vi "Main.vi"() -> ()   [LabVIEW 2026]
doc: "This Continuous Measurement sample project is based on the Queued Message Handler template.\n\nThe Event Handling Loop generates messages based on user interface actions.\n\nThe Message Handling Loop processes messages generated by the Event Handling Loop, or by other messages. There are also Acquisition and Logging message handling loop subVIs, and a chart updating loop."
uses:
  controls/VFD Notifier ctl.ctl
  Settings/Settings.ctl
  Acquisition/Hardware Configuration.ctl
  controls/Durability Test Conditions.ctl
  Logging/Logging Configuration.ctl
  controls/UI Data.ctl
  controls/UI State.ctl
  controls/NotifierAndDataQueue.ctl
  controls/WaveformChartData.ctl
  controls/Abort.vi
  controls/TestCaseTimer.vi
  support/Message Queue/Enqueue Message (Single).vi
  support/Message Queue/Enqueue Message (Array).vi
  <vilib>/Utility/error.llb/Error Cluster From Error Code.vi
  <vilib>/ErrorRing/Error Ring.xnode
  Acquisition/Acquisition.lvlib
  Logging/Logging.lvlib
  Settings/Settings.lvlib
  support/User Event - Stop/User Event - Stop.lvlib
  support/Message Queue/Message Queue.lvlib
  Control/Control.lvlib
panel:
  out "Live Pulley Ratio":dbl format="%#_2g"
  out "Calculated Pulley Ratio":dbl format="%#_2g"
  out "Fault Messages":string[](array[string])
  out "VFD Fault?":bool
  out "Speed (RPM)":dbl
  out "Current (A)":dbl
  out "Voltage (V)":dbl
  in  "Cluster":T1={"Voltage"=0.0, "Current"=0.0, "Motor Speed"=0.0, "Fault"=TRUE, "Fault Messages"=[]}
  in  "Clear Chart":bool
  out "Waveform Chart":T2(graph)
  in  "Tab Control":enum32{"Benchmarking", "Durability"}(tab)
  out "RPM Ramp":bool
  out "Free Air Flow":bool
  out "Press Stable":bool
  out "Press Decay":bool
  out "Status Table":string[][](table)
  out "Test State Timer":dbl(slide) scale=0.0..60.0
  out "INTAKE VALVE POSITION":bool
  out "Air Flow (LPM)":dbl(knob) scale=0.0..100.0
  out "DUT VALVE POSITION":bool
  out "Ambent Temp (F)":dbl(slide) scale=0.0..300.0 scale format="%#_3f"
  out "DUT Motor Current (A)":dbl format="%#_3f"
  out "DUT Temp (F)":dbl(slide) scale=0.0..300.0
  out "DUT Pressure (psi)":dbl(knob) scale=0.0..-15.0
  out "Tank Pressure (psi)":dbl(knob) scale=0.0..-15.0
  out "Drive Motor RPM":dbl(knob) scale=0.0..6000.0 scale format="%#_4f"
  out "DUT Pulley RPM":dbl(knob) scale=0.0..6000.0
  out "Belt Monitor":bool
  out "Status":string
  in  "Exit":bool
  in  "Stop":bool
  in  "Start":bool
  in  "Current Cycle Count":u64
  in  "Tab Control":T3(tab)
  in  "Durability Config File Path":path=path "C:/Users/ROlechna/OneDrive - Dorman Products/Desktop/Book1.csv"
  in  "Motor RPM Target":u16=1000
  in  "Test Selection Box":string(combo)="Benchmarking"
  in  "SKU # or File Name":string
  in  "DUT Motor Direction":bool
  in  "DUT Motor Enable":bool
  in  "Tank Inlet Valve Toggle":bool
  in  "Tank Outlet Valve Toggle":bool
  in  "VFD Enable":bool
  in  "VFD Reset":bool
  # "M1V1-1 Vacuum Pump Tester"
  # "SYSTEM & DUT PROPERTIES"
  # "**Case Timeout = 60s**"
  # "VFD State"
  # "Slot 3 NI 9264"
  # "Benchmarking Test Results"
  # "Durabilty Test Status"
  # "SYSTEM RPM MONITORING"
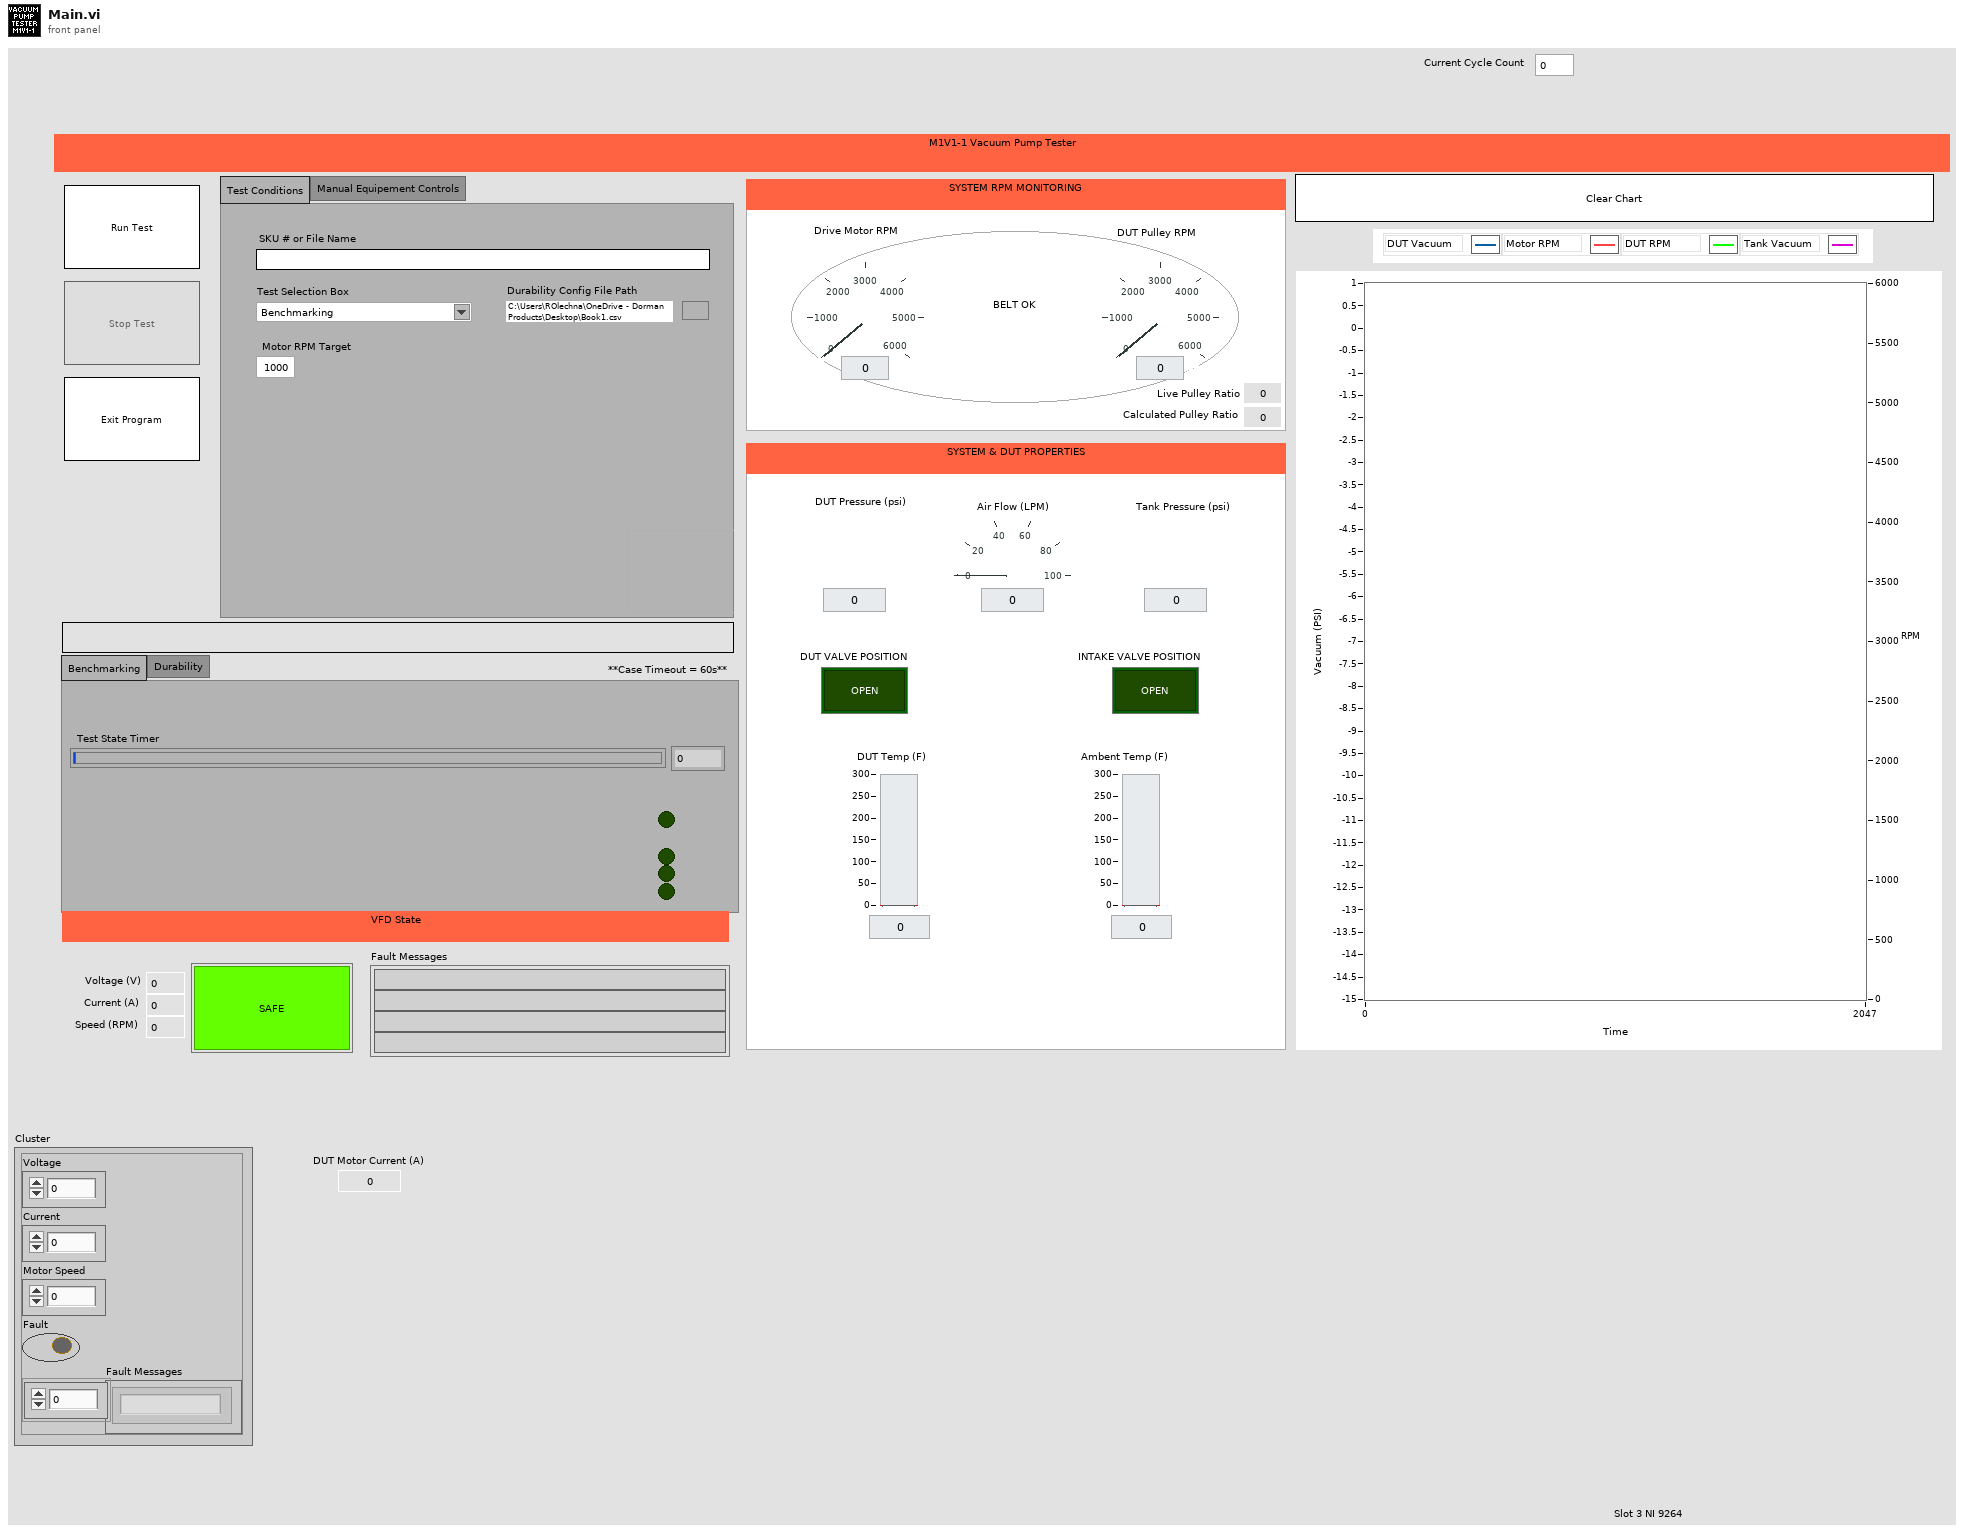
[diagram p1: front panel]
types:
  T1 = typedef "VFD Notifier ctl.ctl" = cluster{"Voltage":dbl, "Current":dbl, "Motor Speed":dbl, "Fault":bool, "Fault Messages":string[]}
  T2 = cluster{"DUT Vacuum":dbl, "Motor RPM":dbl, "DUT RPM":dbl, "Tank Vacuum":dbl}
  T3 = enum32{"Test Conditions", "Manual Equipement Controls"}
  T4 = typedef "NotifierAndDataQueue.ctl" = cluster{"Ai0":dbl, "Ai1":dbl, "Ai2":dbl, "Ai3":dbl, "Ai4":dbl, "Ai5":dbl, "Ai6":dbl, "Ai7":dbl, "Belt Slip?":bool, "P0.1":bool, "P0.2":bool, "P0.3":bool, "P0.4":bool, "P0.5":bool, "P0.6":bool, "P0.7":bool, "2D Numeric Data":dbl[][], "String 2":string, "String 1":string, "Waveform Chart Data":T5, "Live Pulley Ratio":dbl, "Data Table":string[][]}
  T5 = typedef "Settings.lvlib/WaveformChartData.ctl" = cluster{"DUT Vacuum":dbl, "Motor RPM":dbl, "DUT RPM":dbl, "Tank Vacuum":dbl}
  T6 = typedef "UI State.ctl" = enum16{"Idle", "Acquiring and Logging", "Waiting for Exit", "Waiting for Exit (Acq Stopped)", "Waiting for Exit (Log Stopped)", "Waiting for Stop", "Waiting for Stop (Acq Stopped)", "Waiting for Stop (Log Stopped)"}
  T7 = typedef "UI Data.ctl" = cluster{"Start Ref":refnum<vi>, "Trigger Ref":refnum<vi>, "Stop Ref":refnum<vi>, "Settings Ref":refnum<vi>, "Status Ref":refnum<vi>, "Exit Ref":refnum<vi>, "Data Ref":refnum<vi>}
  T8 = typedef "Settings.lvlib/Settings.ctl" = cluster{"Hardware Configuration":T9, "Logging Configuration":T11}
  T9 = typedef "Acquisition.lvlib/Hardware Configuration.ctl" = cluster{"Analog Out array":dbl[], "Initialize Flag":bool, "Saftey Table Display":refnum<vi>, "Torque&Force":waveform(dbl)[][], "Calibration Data":waveform(dbl)[], "2D":dbl[][], "Analog In Task":refnum<k21>, "Digital In Task":refnum<k21>, "Analog Out Task":refnum<k21>, "Digital Out Task":refnum<k21>, "Digital Out Array":bool[], "Current Cycle Count":refnum<vi>, "Cycle Count":u64, "Headers":string[], "Sweep Interval":u64, "Delay":u64, "TestConfigDisplay":refnum<vi>, "50psi Conversion":dbl[], "1245N15 Conversion":dbl[], "MX06F Conversion":dbl[], "# of Test Cycles":u64, "60psi Conversion":dbl[], "100psi Conversion":dbl[], "200psi Conversion":dbl[], "1000psi Conversion":dbl[], "2000psi Conversion":dbl[], "5000psi Conversion":dbl[], "MX09F Conversion":dbl[], "MX19F Conversion":dbl[], "DUT VALVE POSITION":refnum<vi>, "INTAKE VALVE POSITION":refnum<vi>, "Table Control":refnum<vi>, "Table Control":string[][], "Max Vacuum":dbl, "RPM Ramp Ref":refnum<vi>, "Free Air Flow Ref":refnum<vi>, "Press Stable Ref":refnum<vi>, "Press Decay Ref":refnum<vi>, "Pulley Ratio":dbl, "Calculated Pulley Ratio":refnum<vi>, "Durability Test Conditions":T10, "# of Durab Steps":dbl, "manual aquire timer":dbl, "Durability Test Conditions Initial":T10}
  T10 = typedef "Durability Test Conditions.ctl" = cluster{"Step #s":dbl[], "RPMs":dbl[], "Step Durations":dbl[], "Step Delays":dbl[], "Test Cycles":dbl}
  T11 = typedef "Logging.lvlib/Logging Configuration.ctl" = cluster{"Log File Base Path":path, "TDMS File Reference":refnum<k34>, "File Name":string, "Headers To Write":string[]}
  T12 = typedef "Message Queue.lvlib/All Message Queues.ctl" = cluster{"UI":refnum<queue>, "Acquisition":refnum<queue>, "Logging":refnum<queue>, "Control":refnum<queue>, "VFD Control":refnum<queue>}
  T13 = cluster{"DUT Vacuum":dbl, "Motor RPM":dbl, "DUT RPM":dbl, "Tank Vacuum":dbl}[]
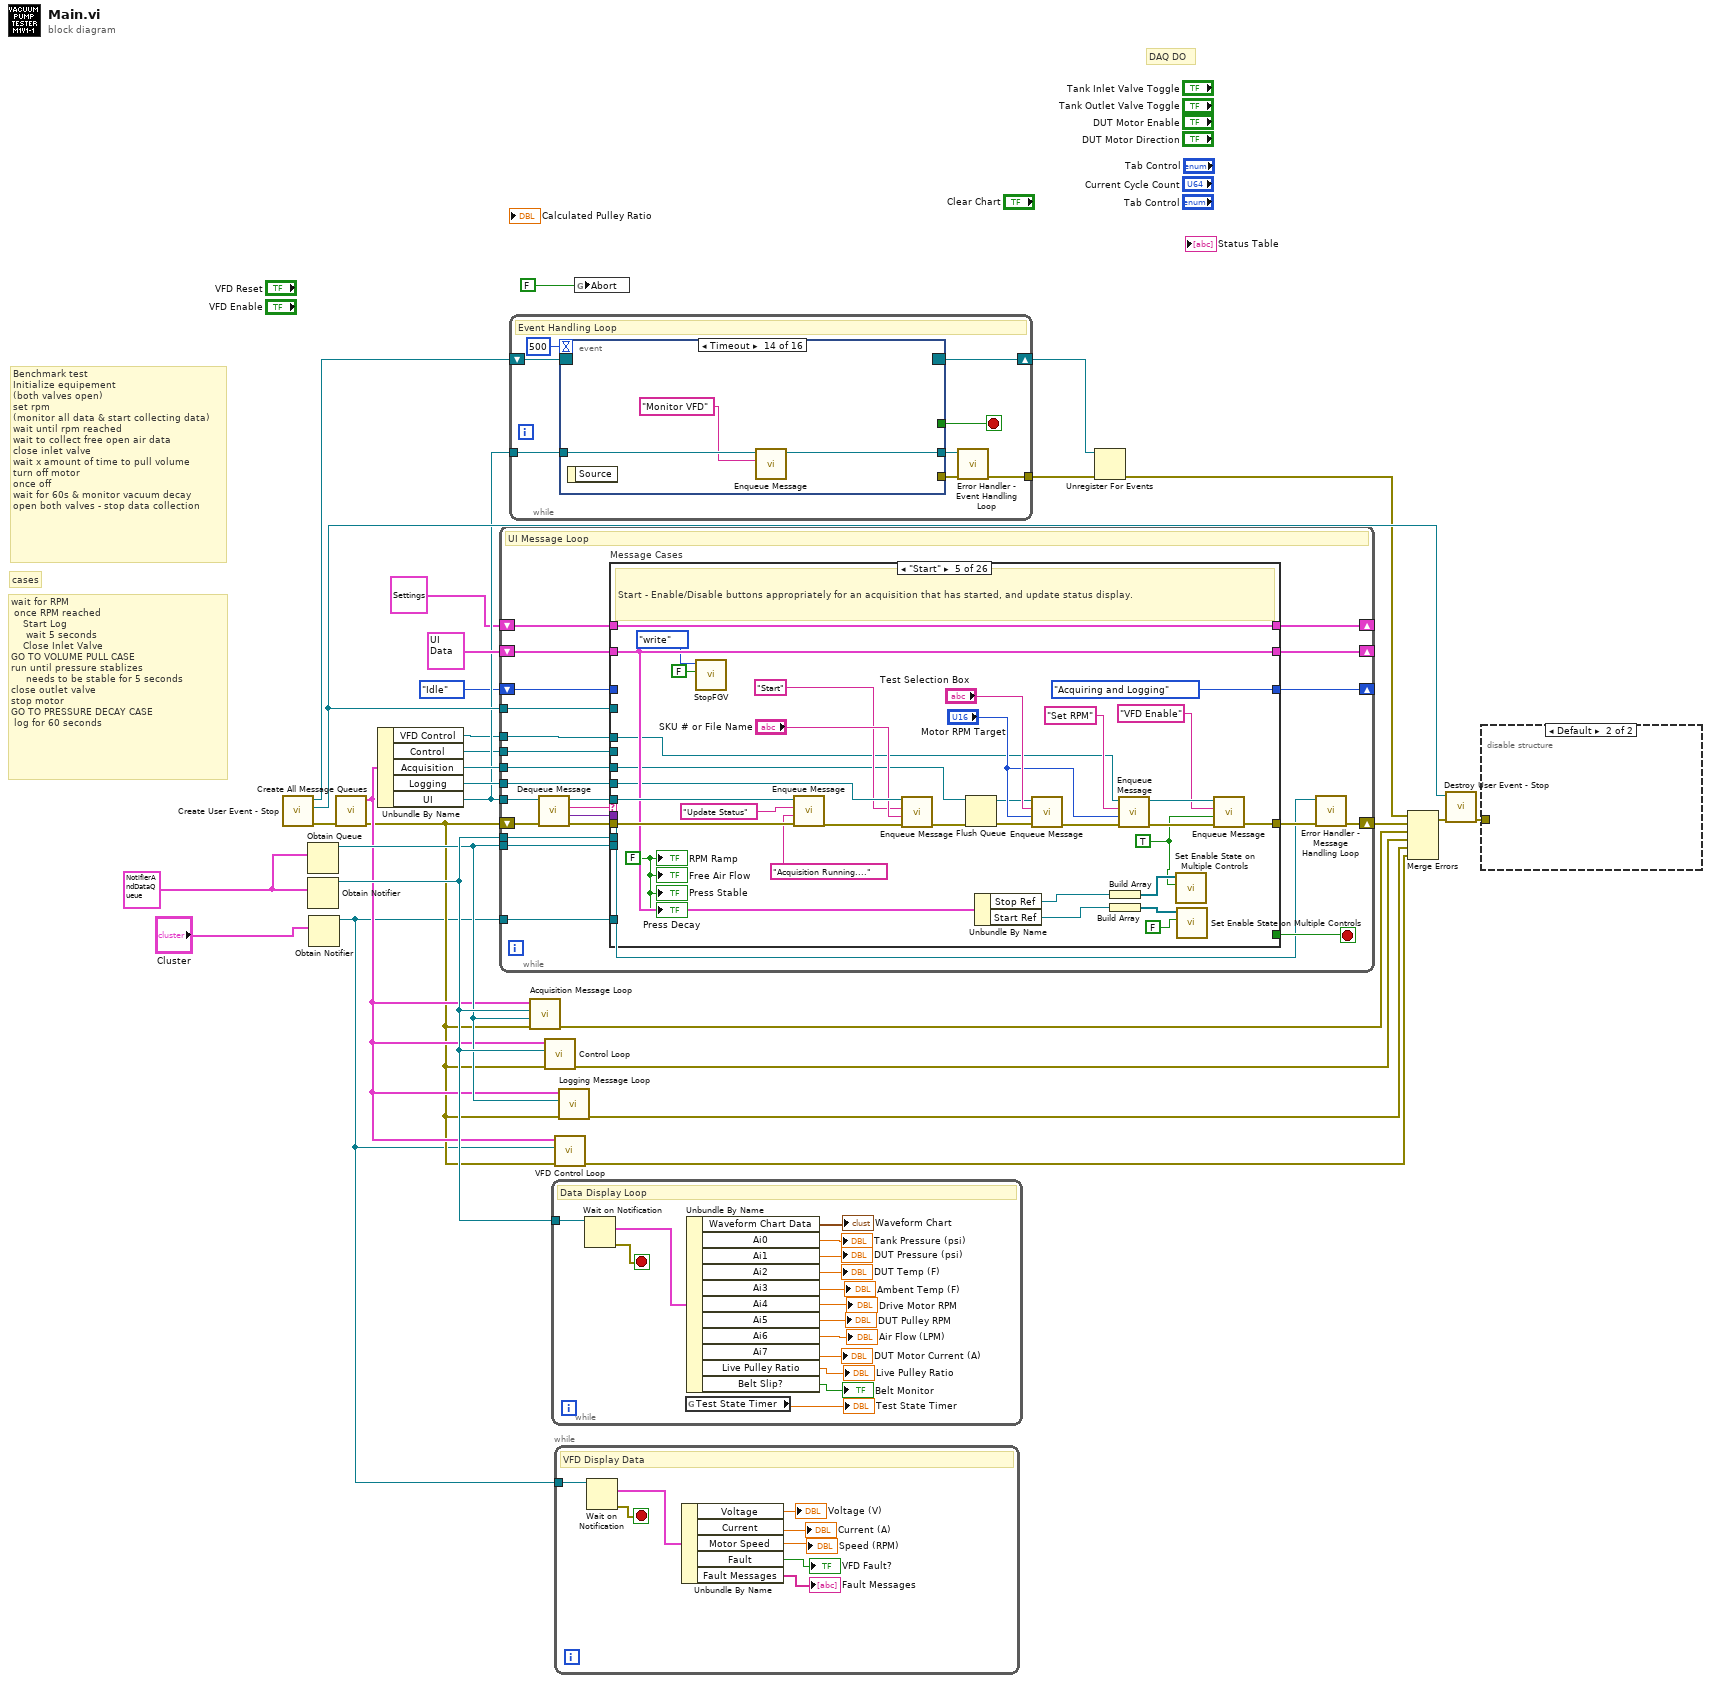
[diagram p0: block diagram]
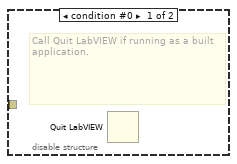
[diagram p2: hidden frame]
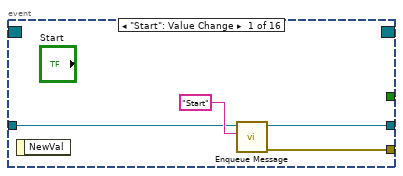
[diagram p3: hidden frame]
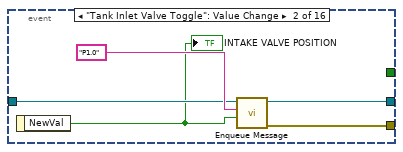
[diagram p4: hidden frame]
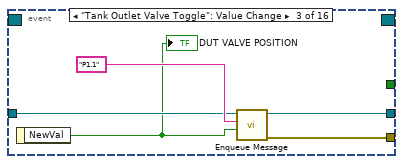
[diagram p5: hidden frame]
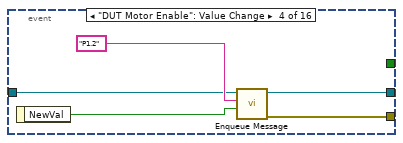
[diagram p6: hidden frame]
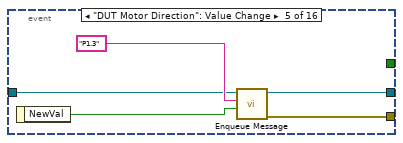
[diagram p7: hidden frame]
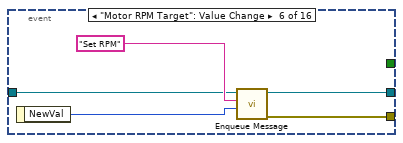
[diagram p8: hidden frame]
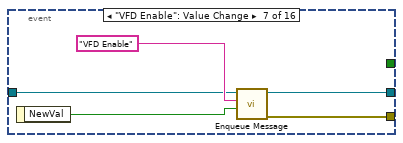
[diagram p9: hidden frame]
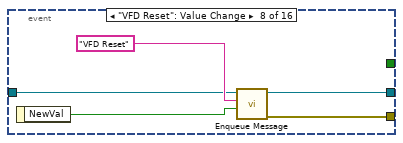
[diagram p10: hidden frame]
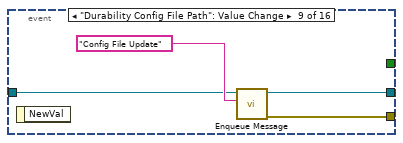
[diagram p11: hidden frame]
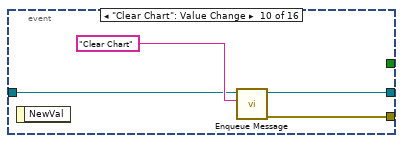
[diagram p12: hidden frame]
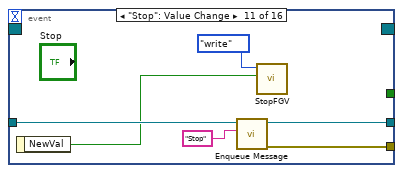
[diagram p13: hidden frame]
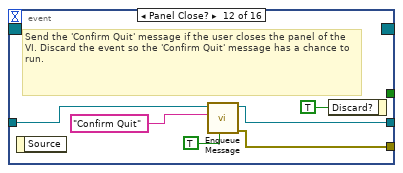
[diagram p14: hidden frame]
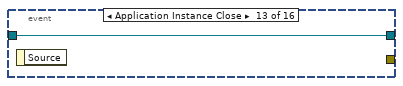
[diagram p15: hidden frame]
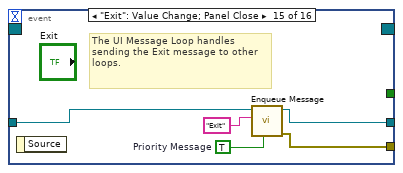
[diagram p16: hidden frame]
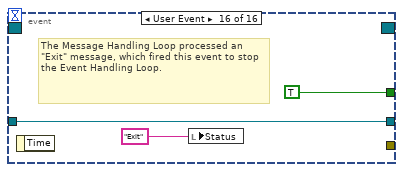
[diagram p17: hidden frame]
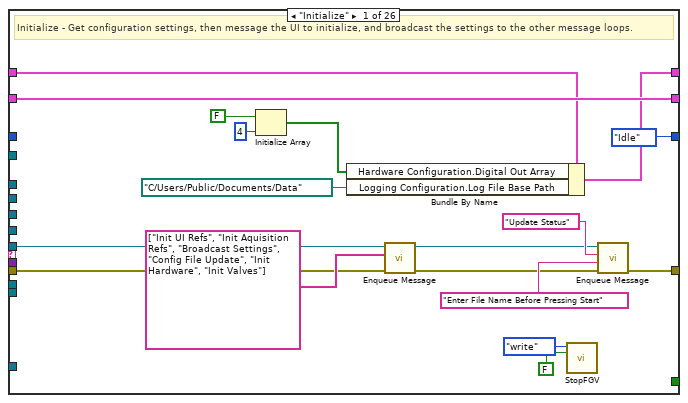
[diagram p18: hidden frame]
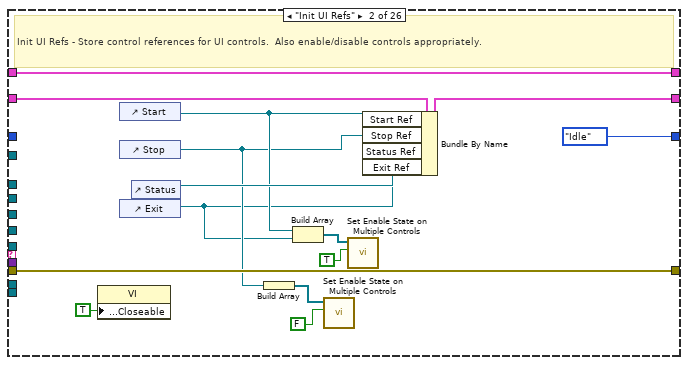
[diagram p19: hidden frame]
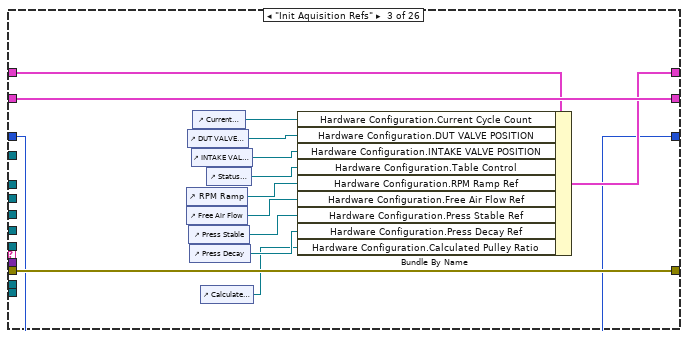
[diagram p20: hidden frame]
diagram:
  w8 = T4 {"Ai0"=0.0, "Ai1"=0.0, "Ai2"=0.0, "Ai3"=0.0, "Ai4"=0.0, "Ai5"=0.0, "Ai6"=0.0, "Ai7"=0.0, "Belt Slip?"=FALSE, "P0.1"=FALSE, "P0.2"=FALSE, "P0.3"=FALSE, "P0.4"=FALSE, "P0.5"=FALSE, "P0.6"=FALSE, "P0.7"=FALSE, "2D Numeric Data"=[], "String 2"="", "String 1"="", "Waveform Chart Data"={"DUT Vacuum"=0.0, "Motor RPM"=0.0, "DUT RPM"=0.0, "Tank Vacuum"=0.0}, "Live Pulley Ratio"=0.0, "Data Table"=[]} ("Waveform")
  # "cases"
  # "wait for RPM\n once RPM reached\n    Start Log\n     wait 5 seconds\n    Close Inlet Valve\nGO TO VOLUME PULL CASE\nrun until pressure stablizes\n     needs to be stable for 5 seconds\nclose outlet valve\nstop motor\nGO TO PRESSURE DECAY CASE\n log for 60 seconds"
  # "Benchmark test\nInitialize equipement\n(both valves open)\nset rpm\n(monitor all data & start collecting data)\nwait until rpm reached\nwait to collect free open air data\nclose inlet valve\nwait x amount of time to pull volume\nturn off motor\nonce off\nwait for 60s & monitor vacuum decay\nopen both valves - stop data collection"
  # "DAQ DO"
  n1 = call "Create User Event - Stop.vi"() -> ("error out"=w23:errorcluster, "User Event - Stop"=w25:refnum<user-event>, "Stop Event Registration Refnum"=w26:refnum<event-registration>)  [unwired: 9 in]
  n2 = Obtain Queue(element data type=w8) -> (queue out=w7:refnum<queue>)  [unwired: 4 in, 2 out]
  n3 = Obtain Notifier(notification data type=w8) -> (notifier out=w9:refnum<notifier>)  [unwired: 3 in, 2 out]
  n4 = Obtain Notifier(notification data type="Cluster") -> (notifier out=w1:refnum<notifier>)  [unwired: 3 in, 2 out]
  n5 = call "Create All Message Queues.vi"("error in (no error)"=w23) -> ("error out"=w5:errorcluster, "Message Queues out"=w6:T12)  [unwired: 9 in]
  n6 = Unbundle By Name(w6) -> ("VFD Control"=w3:refnum<queue>, "Control"=w14:refnum<queue>, "Acquisition"=w19:refnum<queue>, "Logging"=w18:refnum<queue>, "UI"=w17:refnum<queue>)
  n7 = while {
    tunnel: w17 -> [w46]
    tunnel: w25 -> [w51]
    shift-right: [w36] -> w29
    shift-left: w5 -> [w50]
    shift-right: [w45] -> _
    shift-left: T8 {"Hardware Configuration"={"Analog Out array"=[], "Initialize Flag"=FALSE, "Saftey Table Display"=refnum, "Torque&Force"=[], "Calibration Data"=[], "2D"=[], "Analog In Task"="", "Digital In Task"="", "Analog Out Task"="", "Digital Out Task"="", "Digital Out Array"=[], "Current Cycle Count"=refnum, "Cycle Count"=0, "Headers"=[], "Sweep Interval"=0, "Delay"=0, "TestConfigDisplay"=refnum, "50psi Conversion"=[], "1245N15 Conversion"=[], "MX06F Conversion"=[], "# of Test Cycles"=0, "60psi Conversion"=[], "100psi Conversion"=[], "200psi Conversion"=[], "1000psi Conversion"=[], "2000psi Conversion"=[], "5000psi Conversion"=[], "MX09F Conversion"=[], "MX19F Conversion"=[], "DUT VALVE POSITION"=refnum, "INTAKE VALVE POSITION"=refnum, "Table Control"=refnum, "Table Control"=[], "Max Vacuum"=0.0, "RPM Ramp Ref"=refnum, "Free Air Flow Ref"=refnum, "Press Stable Ref"=refnum, "Press Decay Ref"=refnum, "Pulley Ratio"=0.0, "Calculated Pulley Ratio"=refnum, "Durability Test Conditions"={"Step #s"=[], "RPMs"=[], "Step Durations"=[], "Step Delays"=[], "Test Cycles"=0.0}, "# of Durab Steps"=0.0, "manual aquire timer"=0.0, "Durability Test Conditions Initial"={"Step #s"=[], "RPMs"=[], "Step Durations"=[], "Step Delays"=[], "Test Cycles"=0.0}}, "Logging Configuration"={"Log File Base Path"=path "", "TDMS File Reference"=refnum, "File Name"="", "Headers To Write"=[]}} ("Settings") -> [w44]
    shift-right: [w42] -> _
    shift-left: T7 {"Start Ref"=refnum, "Trigger Ref"=refnum, "Stop Ref"=refnum, "Settings Ref"=refnum, "Status Ref"=refnum, "Exit Ref"=refnum, "Data Ref"=refnum} ("Measurement UI Controls") -> [w43]
    tunnel: w19 -> [w41]
    tunnel: w18 -> [w40]
    tunnel: w9 -> [w39]
    tunnel: w7 -> [w38]
    shift-right: [w33] -> _
    shift-left: UI_State."Idle" ("UI State") -> [w34]
    tunnel: w14 -> [w32]
    tunnel: w3 -> [w31]
    tunnel: w1 -> [w30]
    stop <- w52 stop-if-true
    # "UI Message Loop"
    n8 = call "Dequeue Message.vi"("error in (no error)"=w50, "Message Queue"=w46) -> ("error out"=w49:errorcluster, "Message Data"=w47:variant, "Message"=w48:string, "dup Message Queue"=w35:refnum<queue>)  [unwired: 6 in]
    n9 = case "Message Cases" shown="\"Start\"" w48 {
      selector: w48 -> [_ _ _ _ _ _ _ _ _ _ _ _ _ _ _ _ _ _ _ _ _ _ _ _ _ w420]
      tunnel: w35 -> [w66 _ _ _ w140 _ _ w161 _ _ _ _ _ w241 w251 w276 _ _ _ _ _ _ w360 w370 w408 _]
      tunnel: w49 -> [w65 w84 w98 w106 w139 w146 w155 w171 w179 w188 w197 w206 w215 w240 w253 w278 w306 w321 w329 w336 w341 w349 w364 w369 w413 _]
      tunnel: [w53 w84 w98 w107 w120 w149 w158 w173 w182 w191 w200 w209 w218 w224 w252 w277 w301 w315 w328 w335 w341 w348 w355 w368 w414 w421] -> w37
      tunnel: [_ _ _ _ _ _ _ _ _ _ _ _ _ _ _ _ _ _ _ _ _ _ _ _ TRUE _] -> w52
      tunnel: w47 -> [_ _ _ w105 _ w141 w150 _ w174 w183 w193 w202 w211 _ _ _ _ _ _ _ _ _ w363 _ _ _]
      tunnel: w51 -> [_ _ _ _ _ _ _ _ _ _ _ _ _ _ _ _ _ _ _ _ _ _ _ _ w412 _]
      tunnel: [w63 w83 w95 w102 w128 w148 w157 w172 w181 w190 w199 w208 w217 w239 w257 w282 w305 w323 w331 w338 w344 w353 w366 w373 w410 w423] -> w45
      tunnel: w44 -> [w54 w83 w96 w102 w128 w148 w157 w172 w181 w190 w199 w208 w217 w239 w257 w282 w305 w323 w331 w338 w344 w353 w366 w373 w410 w423]
      tunnel: w43 -> [w68 w82 w97 w101 w136 w147 w156 w165 w180 w189 w198 w207 w216 w236 w256 w281 w308 w322 w330 w337 w343 w352 w365 w372 w409 w422]
      tunnel: [w68 w81 w97 w101 w136 w147 w156 w165 w180 w189 w198 w207 w216 w236 w256 w281 w308 w322 w330 w337 w343 w352 w365 w372 w409 w422] -> w42
      tunnel: w41 -> [_ _ _ _ w108 _ _ w168 _ _ _ _ _ w222 _ _ w303 w320 _ _ _ w347 _ _ w401 _]
      tunnel: w40 -> [_ _ _ _ w130 _ _ _ _ _ _ _ _ w221 _ _ _ _ _ _ _ _ _ _ w400 _]
      tunnel: w39 -> [_ _ _ _ _ _ _ _ _ _ _ _ _ _ _ _ _ _ _ _ _ _ _ _ w407 _]
      tunnel: w38 -> [_ _ _ _ _ _ _ _ _ _ _ _ _ _ _ _ _ _ _ _ _ _ _ _ w404 _]
      tunnel: w34 -> [_ _ w94 w99 _ w143 w152 _ w176 w185 w194 w203 w212 w226 w255 w280 w307 w316 w324 w334 w342 w350 w354 w371 _ w419]
      tunnel: [UI_State."Idle" ("UI State") UI_State."Idle" ("UI State") w94 w99 UI_State."Acquiring and Logging" ("UI State") w143 w152 UI_State."Acquiring and Logging" ("UI State") w176 w185 w194 w203 w212 w225 w254 w279 w307 w316 w324 w334 w342 w350 w354 w367 UI_State."Idle" ("UI State") w419] -> w33
      tunnel: w32 -> [_ _ _ _ _ w142 w151 _ w175 w184 _ _ _ w223 _ _ w302 w318 w327 _ _ _ _ _ w402 _]
      tunnel: w31 -> [_ _ _ _ w112 _ _ _ _ _ w192 w201 w210 w219 _ _ _ _ _ w332 _ _ _ _ w398 _]
      tunnel: w30 -> [_ _ _ _ _ _ _ _ _ _ _ _ _ _ _ _ _ _ _ _ _ _ _ _ w395 _]
      frame "Initialize" {
        # "Initialize - Get configuration settings, then message the UI to initialize, and broadcast the settings to the other message loops."
        n10 = Initialize Array(FALSE, 4 ("dimension size")) -> (w57:bool[])
        n11 = Bundle By Name(cluster=w54, "Hardware Configuration.Digital Out Array"=w57, "Logging Configuration.Log File Base Path"=path "C:/Users/Public/Documents/Data") -> (w63:T8)
        n12 = call-poly "Enqueue Message.vi"("error in (no error)"=w65, "Message Array"=string[] ["Init UI Refs", "Init Aquisition Refs", "Broadcast Settings", "Config File Update", "Init Hardware", "Init Valves"] ("Message"), "Message Queue"=w66) -> ("error out"=w61:errorcluster, "dup Message Queue"=w62:refnum<queue>)  [unwired: 7 in]
        n13 = call "StopFGV.vi"("STOP"=FALSE, "Enum"=enum16{"init", "write", "read"}."write") -> ()  [unwired: 8 in, 2 out]
        n14 = call-poly "Enqueue Message.vi"("error in (no error)"=w61, "Message Data"="Enter File Name Before Pressing Start" ("Ready..."), "Message"="Update Status", "Message Queue"=w62) -> ("error out"=w53:errorcluster)  [unwired: 6 in, 1 out]
      }
      frame "Init UI Refs" {
        # "Init UI Refs - Store control references for UI controls.  Also enable/disable controls appropriately."
        n15 = property class="VI"("Front Panel.Closeable"=TRUE ("Front Panel Window:Closeable")) -> ()  [unwired: 2 in, 2 out]
        n16 = control-ref of="Start"() -> (w73:refnum<vi>)
        n17 = control-ref of="Stop"() -> (w72:refnum<vi>)
        n18 = control-ref of="Exit"() -> (w71:refnum<vi>)
        n19 = control-ref of="Status"() -> (w78:refnum<vi>)
        n20 = Build Array(w72) -> (w77:refnum<vi>[])
        n21 = Build Array(w73, w71) -> (w75:refnum<vi>[])
        n22 = call "Set Enable State on Multiple Controls.vi"("Enable?"=FALSE, "Controls"=w77) -> ()  [unwired: 10 in]
        n23 = call "Set Enable State on Multiple Controls.vi"("Enable?"=TRUE, "Controls"=w75) -> ()  [unwired: 10 in]
        n24 = Bundle By Name(cluster=w82, "Start Ref"=w73, "Stop Ref"=w72, "Status Ref"=w78, "Exit Ref"=w71) -> (w81:T7)
      }
      frame "Init Aquisition Refs" {
        n25 = control-ref of="RPM Ramp"() -> (w89:refnum<vi>)
        n26 = control-ref of="Free Air Flow"() -> (w88:refnum<vi>)
        n27 = control-ref of="DUT VALVE POSITION"() -> (w92:refnum<vi>)
        n28 = control-ref of="Press Stable"() -> (w87:refnum<vi>)
        n29 = control-ref of="Press Decay"() -> (w86:refnum<vi>)
        n30 = control-ref of="INTAKE VALVE POSITION"() -> (w91:refnum<vi>)
        n31 = control-ref of="Current Cycle Count"() -> (w93:refnum<vi>)
        n32 = control-ref of="Calculated Pulley Ratio"() -> (w85:refnum<vi>)
        n33 = control-ref of="Status Table"() -> (w90:refnum<vi>)
        n34 = Bundle By Name(cluster=w96, "Hardware Configuration.Current Cycle Count"=w93, "Hardware Configuration.DUT VALVE POSITION"=w92, "Hardware Configuration.INTAKE VALVE POSITION"=w91, "Hardware Configuration.Table Control"=w90, "Hardware Configuration.RPM Ramp Ref"=w89, "Hardware Configuration.Free Air Flow Ref"=w88, "Hardware Configuration.Press Stable Ref"=w87, "Hardware Configuration.Press Decay Ref"=w86, "Hardware Configuration.Calculated Pulley Ratio"=w85) -> (w95:T8)
      }
      frame "Update Status" {
        # "Update Display - Convert the message data to a string to display in the Status indicator."
        n35 = Variant To Data(error in=w106, type="", Variant=w105) -> (data=→"Status":string, error out=w103:errorcluster)
        n36 = Merge Errors(w103) -> (w107:errorcluster)
      }
      frame "Start" {
        w121 = FALSE
        w114 = TRUE ("Enable?")
        # "Start - Enable/Disable buttons appropriately for an acquisition that has started, and update status display."
        n37 = call "StopFGV.vi"("STOP"=FALSE, "Enum"=enum16{"init", "write", "read"}."write") -> ()  [unwired: 8 in, 2 out]
        n38 = call-poly "Enqueue Message.vi"("error in (no error)"=w139, "Message Data"="Acquisition Running...." ("Waiting for trigger"), "Message"="Update Status", "Message Queue"=w140) -> ("error out"=w131:errorcluster)  [unwired: 6 in, 1 out]
        n39 = call-poly "Enqueue Message.vi"("error in (no error)"=w131, "Message Data"="SKU # or File Name", "Message"="Start", "Message Queue"=w130) -> ("error out"=w111:errorcluster)  [unwired: 6 in, 1 out]
        n40 = Flush Queue(queue=w108, error in (no error)=w111) -> (queue out=w109:refnum<queue>, error out=w110:errorcluster)  [unwired: 1 out]
        n41 = Unbundle By Name(w136) -> ("Stop Ref"=w127:refnum<vi>, "Start Ref"=w132:refnum<vi>)
        n42 = call-poly "Enqueue Message.vi"("error in (no error)"=w110, "Message Data"="Motor RPM Target", "Message"="Test Selection Box", "Message Queue"=w109) -> ("error out"=w119:errorcluster)  [unwired: 6 in, 1 out]
        n43 = Build Array(w127) -> (w133:refnum<vi>[])
        n44 = Build Array(w132) -> (w134:refnum<vi>[])
        n45 = call-poly "Enqueue Message.vi"("error in (no error)"=w119, "Message Data"="Motor RPM Target", "Message"="Set RPM", "Message Queue"=w112) -> ("error out"=w118:errorcluster, "dup Message Queue"=w117:refnum<queue>)  [unwired: 6 in]
        n46 = call "Set Enable State on Multiple Controls.vi"("Enable?"=w114, "Controls"=w133) -> ()  [unwired: 10 in]
        n47 = call "Set Enable State on Multiple Controls.vi"("Enable?"=FALSE, "Controls"=w134) -> ()  [unwired: 10 in]
        n48 = call-poly "Enqueue Message.vi"("error in (no error)"=w118, "Message Data"=w114, "Message"="VFD Enable", "Message Queue"=w117) -> ("error out"=w120:errorcluster)  [unwired: 6 in, 1 out]
        "RPM Ramp" <- w121
        "Free Air Flow" <- w121
        "Press Stable" <- w121
        "Press Decay" <- w121
      }
      frame "P1.0" {
        # "Force Trigger - send a message to the Logging message loop to start logging."
        n49 = call-poly "Enqueue Message.vi"("error in (no error)"=w146, "Message Data"=w141, "Message"="P1.0", "Message Queue"=w142) -> ("error out"=w145:errorcluster)  [unwired: 6 in, 1 out]
        n50 = Merge Errors(w145) -> (w149:errorcluster)
      }
      frame "P1.1" {
        # "Force Trigger - send a message to the Logging message loop to start logging."
        n51 = call-poly "Enqueue Message.vi"("error in (no error)"=w155, "Message Data"=w150, "Message"="P1.1", "Message Queue"=w151) -> ("error out"=w154:errorcluster)  [unwired: 6 in, 1 out]
        n52 = Merge Errors(w154) -> (w158:errorcluster)
      }
      frame "Manual Acquire" {
        # "Force Trigger - send a message to the Logging message loop to start logging."
        n53 = Unbundle By Name(w165) -> ("Stop Ref"=w164:refnum<vi>)
        n54 = Build Array(w164) -> (w166:refnum<vi>[])
        n55 = call-poly "Enqueue Message.vi"("error in (no error)"=w171, "Message"="Start", "Message Queue"=w168) -> ("error out"=w163:errorcluster)  [unwired: 7 in, 1 out]
        n56 = call "Set Enable State on Multiple Controls.vi"("Enable?"=TRUE, "Controls"=w166) -> ()  [unwired: 10 in]
        n57 = call-poly "Enqueue Message.vi"("error in (no error)"=w163, "Message Data"="Manually Acquiring...." ("Message"), "Message"="Update Status", "Message Queue"=w161) -> ("error out"=w162:errorcluster)  [unwired: 6 in, 1 out]
        n58 = Merge Errors(w162) -> (w173:errorcluster)
      }
      frame "P1.2" {
        # "Force Trigger - send a message to the Logging message loop to start logging."
        n59 = call-poly "Enqueue Message.vi"("error in (no error)"=w179, "Message Data"=w174, "Message"="P1.2", "Message Queue"=w175) -> ("error out"=w178:errorcluster)  [unwired: 6 in, 1 out]
        n60 = Merge Errors(w178) -> (w182:errorcluster)
      }
      frame "P1.3" {
        # "Force Trigger - send a message to the Logging message loop to start logging."
        n61 = call-poly "Enqueue Message.vi"("error in (no error)"=w188, "Message Data"=w183, "Message"="P1.3", "Message Queue"=w184) -> ("error out"=w187:errorcluster)  [unwired: 6 in, 1 out]
        n62 = Merge Errors(w187) -> (w191:errorcluster)
      }
      frame "Set RPM" {
        # "Force Trigger - send a message to the Logging message loop to start logging."
        n63 = call-poly "Enqueue Message.vi"("error in (no error)"=w197, "Message Data"=w193, "Message"="Set RPM", "Message Queue"=w192) -> ("error out"=w196:errorcluster)  [unwired: 6 in, 1 out]
        n64 = Merge Errors(w196) -> (w200:errorcluster)
      }
      frame "VFD Enable" {
        # "Force Trigger - send a message to the Logging message loop to start logging."
        n65 = call-poly "Enqueue Message.vi"("error in (no error)"=w206, "Message Data"=w202, "Message"="VFD Enable", "Message Queue"=w201) -> ("error out"=w205:errorcluster)  [unwired: 6 in, 1 out]
        n66 = Merge Errors(w205) -> (w209:errorcluster)
      }
      frame "VFD Reset" {
        # "Force Trigger - send a message to the Logging message loop to start logging."
        n67 = call-poly "Enqueue Message.vi"("error in (no error)"=w215, "Message Data"=w211, "Message"="VFD Reset", "Message Queue"=w210) -> ("error out"=w214:errorcluster)  [unwired: 6 in, 1 out]
        n68 = Merge Errors(w214) -> (w218:errorcluster)
      }
      frame "Stop" {
        # "Stop - Enable/Disable buttons appropriately for an acquisition that has stopped, and update status display."
        n69 = Unbundle By Name(w236) -> ("Stop Ref"=w227:refnum<vi>, "Start Ref"=w231:refnum<vi>, "Exit Ref"=w230:refnum<vi>, "Settings Ref"=w229:refnum<vi>)
        n70 = Build Array(w219, w223, w222, w221) -> (w220:refnum<queue>[])
        n71 = Build Array(w231, w230, w229) -> (w234:refnum<vi>[])
        n72 = call-poly "Enqueue Message.vi"("error in (no error)"=w240, "Message Data"="Stop Button Pressed" ("Ready..."), "Message"="Update Status", "Message Queue"=w241) -> ("error out"=w228:errorcluster)  [unwired: 6 in, 1 out]
        n73 = Build Array(w227) -> (w233:refnum<vi>[])
        n74 = call "Set Enable State on Multiple Controls.vi"("Enable?"=TRUE, "Controls"=w234) -> ()  [unwired: 10 in]
        n75 = call "Set Enable State on Multiple Controls.vi"("Enable?"=FALSE, "Controls"=w233) -> ()  [unwired: 10 in]
        n76 = for {
          tunnel: w228 -> [w244]
          tunnel: [w247] -> w224
          tunnel: w220 -> [w245] mode=indexing
          n77 = Flush Queue(queue=w245, error in (no error)=w244) -> (queue out=w242:refnum<queue>, error out=w243:errorcluster)  [unwired: 1 out]
          n78 = call-poly "Enqueue Message.vi"("Priority Message? (F)"=TRUE, "error in (no error)"=w243, "Message"="Stop", "Message Queue"=w242) -> ("error out"=w247:errorcluster)  [unwired: 6 in, 1 out]
        }
        n79 = case shown="Default" w226 {
          selector: w226 -> [_ w250]
          tunnel: [UI_State."Waiting for Stop" ("UI State") w250] -> w225
          frame Default {
          }
          frame "Waiting for Exit" {
          }
        }
      }
      frame "Acquisition Stopped" {
        # "Logic for determining what action to take when the acquisition has stopped."
        n80 = case shown="\"Waiting for Stop\", \"Waiting for Stop (Acq Stopped)\"" w255 {
          selector: w255 -> [w259 _ _ _ _]
          tunnel: [w259 UI_State."Waiting for Exit (Acq Stopped)" ("UI State") UI_State."Waiting for Stop (Acq Stopped)" ("UI State") UI_State."Idle" ("UI State") UI_State."Idle" ("UI State")] -> w254
          tunnel: w253 -> [w258 w260 w262 w268 w274]
          tunnel: [w258 w260 w262 w267 w273] -> w252
          tunnel: w251 -> [_ _ _ w266 w272]
          frame Default {
          }
          frame "Waiting for Exit", "Waiting for Exit (Acq Stopped)" {
          }
          frame "Waiting for Stop", "Waiting for Stop (Acq Stopped)" {
          }
          frame "Waiting for Exit (Log Stopped)" {
            # "If we are waiting to exit, and the logging has already stopped, then the \"Acquisition Stopped\" message indicates that it is time to exit."
            n81 = call-poly "Enqueue Message.vi"("Priority Message? (F)"=TRUE, "error in (no error)"=w268, "Message"="Exit", "Message Queue"=w266) -> ("error out"=w267:errorcluster)  [unwired: 6 in, 1 out]
          }
          frame "Waiting for Stop (Log Stopped)" {
            # "If we are waiting to stop, and the logging has already stopped, then the \"Acquisition Stopped\" message indicates that it is time to stop."
            n82 = call-poly "Enqueue Message.vi"("error in (no error)"=w274, "Message Data"="Ready..." ("Message"), "Message"="Update Status", "Message Queue"=w272) -> ("error out"=w273:errorcluster)  [unwired: 6 in, 1 out]
          }
        }
      }
      frame "Logging Stopped" {
        # "Logic for determining what action to take when the logging has stopped."
        n83 = case shown="\"Waiting for Exit\", \"Waiting for Exit (Log Stopped)\"" w280 {
          selector: w280 -> [w284 _ _ _ _]
          tunnel: [w284 UI_State."Waiting for Exit (Log Stopped)" ("UI State") UI_State."Waiting for Stop (Log Stopped)" ("UI State") UI_State."Idle" ("UI State") UI_State."Idle" ("UI State")] -> w279
          tunnel: w278 -> [w283 w285 w287 w293 w299]
          tunnel: [w283 w285 w287 w292 w298] -> w277
          tunnel: w276 -> [_ _ _ w291 w297]
          frame Default {
          }
          frame "Waiting for Exit", "Waiting for Exit (Log Stopped)" {
          }
          frame "Waiting for Stop", "Waiting for Stop (Log Stopped)" {
          }
          frame "Waiting for Exit (Acq Stopped)" {
            # "If we are waiting to exit, and the acquisition has already stopped, then the \"Logging Stopped\" message indicates that it is time to exit."
            n84 = call-poly "Enqueue Message.vi"("Priority Message? (F)"=TRUE, "error in (no error)"=w293, "Message"="Exit", "Message Queue"=w291) -> ("error out"=w292:errorcluster)  [unwired: 6 in, 1 out]
          }
          frame "Waiting for Stop (Acq Stopped)" {
            # "If we are waiting to stop, and the acquisition has already stopped, then the \"Logging Stopped\" message indicates that it is time to stop."
            n85 = call-poly "Enqueue Message.vi"("error in (no error)"=w299, "Message Data"="Ready..." ("Message"), "Message"="Update Status", "Message Queue"=w297) -> ("error out"=w298:errorcluster)  [unwired: 6 in, 1 out]
          }
        }
      }
      frame "Broadcast settings" {
        # "Send the 'Update Settings' message to the Logging and Acquisition message loops."
        n86 = Build Array(w302, w303) -> (w304:refnum<queue>[])
        n87 = for {
          tunnel: w306 -> [w310]
          tunnel: [w311] -> w301
          tunnel: w305 -> [w314]
          tunnel: w304 -> [w312] mode=indexing
          n88 = Unbundle By Name(w314) -> ("Hardware Configuration"=w309:T9)
          n89 = call-poly "Enqueue Message.vi"("error in (no error)"=w310, "Message Data"=w309, "Message"="Update Settings", "Message Queue"=w312) -> ("error out"=w311:errorcluster)  [unwired: 6 in, 1 out]
        }
      }
      frame "Init Hardware" {
        w317 = "Start" ("Message")
        n90 = call-poly "Enqueue Message.vi"("error in (no error)"=w321, "Message"=w317, "Message Queue"=w320) -> ("error out"=w319:errorcluster)  [unwired: 7 in, 1 out]
        n91 = call-poly "Enqueue Message.vi"("error in (no error)"=w319, "Message"=w317, "Message Queue"=w318) -> ("error out"=w315:errorcluster)  [unwired: 7 in, 1 out]
      }
      frame "Init Valves" {
        n92 = call-poly "Enqueue Message.vi"("error in (no error)"=w329, "Message Data Array"=bool[] [FALSE, FALSE], "Message Array"=string[] ["P1.0", "P1.1"], "Message Queue"=w327) -> ("error out"=w328:errorcluster)  [unwired: 6 in, 1 out]
      }
      frame "Monitor VFD" {
        n93 = call-poly "Enqueue Message.vi"("error in (no error)"=w336, "Message"="Monitor VFD", "Message Queue"=w332) -> ("error out"=w335:errorcluster)  [unwired: 7 in, 1 out]
      }
      frame "Clear Chart" {
        n94 = property on="Waveform Chart" class="WFChart (strict)"("Value"=T2 {"DUT Vacuum"=0.0, "Motor RPM"=0.0, "DUT RPM"=0.0, "Tank Vacuum"=0.0} ("Waveform Chart"), "History Data"=T13 []) -> ()  [unwired: 2 in, 2 out]
      }
      frame "Config File Update" {
        n95 = call "Durability Test Conditions Grabber.vi"("file path"="Durability Config File Path") -> ("Durability Test Conditions"=w345:T10)  [unwired: 10 in]
        n96 = call-poly "Enqueue Message.vi"("error in (no error)"=w349, "Message Data"=w345, "Message"="Config File Update", "Message Queue"=w347) -> ("error out"=w348:errorcluster)  [unwired: 6 in, 1 out]
      }
      frame "Error" {
        # "Error - Check the error message data and respond accordingly. This message is sent by the \"Error Handler\" VIs at the end of each loop in this application."
        n97 = Variant To Data(error in=w364, type=errorcluster {"status"=FALSE, "code"=0, "source"=""} ("error out"), Variant=w363) -> (data=w361:errorcluster, error out=w357:errorcluster)
        n98 = call <vilib>:"Simple Error Handler.vi"("error in (no error)"=w361) -> ()  [unwired: 4 in, 5 out]
        n99 = call-poly "Enqueue Message.vi"("Priority Message? (F)"=TRUE, "Message"="Exit", "Message Queue"=w360) -> ("error out"=w356:errorcluster)  [unwired: 7 in, 1 out]
        n100 = Merge Errors(w356, w357) -> (w355:errorcluster)
      }
      frame "Confirm Quit" {
        # "Confirm Quit - Message that can confirm whether or not the user wants to exit the application."
        n101 = case shown="\"Acquiring and Logging\"" w371 {
          tunnel: w370 -> [w378 w384]
          tunnel: w369 -> [w377 w382]
          tunnel: [w374 w381] -> w368
          tunnel: [UI_State."Idle" ("UI State") w380] -> w367
          frame Default {
            # "If 'Confirm Quit' comes in while the system is idle, there is no need for a confirmation message."
            n102 = call-poly "Enqueue Message.vi"("Priority Message? (F)"=TRUE, "error in (no error)"=w377, "Message"="Exit", "Message Queue"=w378) -> ("error out"=w374:errorcluster)  [unwired: 6 in, 1 out]
          }
          frame "Acquiring and Logging" {
            n103 = Two Button Dialog(message="Are you sure you want to quit while the acquisition is running?" ("Confirm Quit Message"), 1:"No" ("No"), 2:"Yes" ("Yes")) -> (T button?=w383:bool)
            n104 = case shown="True" w383 {
              tunnel: w384 -> [_ w394]
              tunnel: w382 -> [w388 w393]
              tunnel: [w388 w392] -> w381
              tunnel: [UI_State."Acquiring and Logging" ("UI State") UI_State."Waiting for Exit" ("UI State")] -> w380
              frame False {
                # "User did not want to quit."
              }
              frame True {
                n105 = call-poly "Enqueue Message.vi"("error in (no error)"=w393, "Message"="Stop", "Message Queue"=w394) -> ("error out"=w392:errorcluster)  [unwired: 7 in, 1 out]
              }
            }
          }
        }
      }
      frame "Exit" {
        # "Stop the VI"
        # "Exit - Fire the User Event to stop the Event Handling Loop.  Also send Exit messages to the Acquisition and Logging loops."
        n106 = Release Queue(queue=w408, error in (no error)=w413) -> (error out=w406:errorcluster)  [unwired: 1 in, 2 out]
        n107 = Build Array(w398, w402, w401, w400) -> (w399:refnum<queue>[])
        n108 = Release Notifier(notifier=w407, error in (no error)=w406) -> (error out=w405:errorcluster)  [unwired: 1 in, 2 out]
        n109 = Release Queue(queue=w404, error in (no error)=w405) -> (error out=w396:errorcluster)  [unwired: 1 in, 2 out]
        n110 = Release Notifier(notifier=w395, error in (no error)=w396) -> (error out=w397:errorcluster)  [unwired: 1 in, 2 out]
        n111 = for {
          tunnel: w399 -> [w418] mode=indexing
          n112 = call-poly "Enqueue Message.vi"("Priority Message? (F)"=TRUE, "Message"="Exit", "Message Queue"=w418) -> ()  [unwired: 7 in, 2 out]
        }
        n113 = call "Fire User Event - Stop.vi"("User Event - Stop"=w412) -> ("error out"=w411:errorcluster)  [unwired: 10 in]
        n114 = Merge Errors(w411, w397) -> (w414:errorcluster)
      }
      frame Default {
        # "'Default' case only runs if there is a message that isn't defined in any of the other cases.  Output a programming error."
        n115 = xnode "Error Ring"("parameter 0"=w420) -> ("error out"=w421:errorcluster)
      }
    }
    n116 = call "Error Handler - Message Handling Loop.vi"("error in (no error)"=w37, "Message Queue"=w35) -> ("dup error in"=w36:errorcluster)  [unwired: 8 in, 1 out]
  }
  n117 = while {
    tunnel: w17 -> [w437]
    tunnel: [w432] -> w28
    shift-right: [w436] -> w21
    shift-left: w26 -> [w438]
    stop <- w435 stop-if-true
    # "Event Handling Loop"
    n118 = event shown="[13] Timeout" {
      selector: w438 -> [_ _ _ _ _ _ _ _ _ _ _ _ _ _ _ _]
      dyn-events: [_ _ _ _ _ _ _ _ _ _ _ _ _ _ _ _] -> w436
      timeout: 500 -> [_ _ _ _ _ _ _ _ _ _ _ _ _ _ _ _]
      tunnel: [_ _ _ _ _ _ _ _ _ _ _ _ _ _ _ TRUE ("Discard?")] -> w435
      tunnel: w437 -> [w440 w445 w450 w455 w460 w465 w470 w475 w479 w483 w490 w497 w498 w501 w503 w507]
      tunnel: [w442 w447 w452 w457 w462 w467 w472 w477 w481 w485 w489 w492 _ _ w506 _] -> w433
      tunnel: [w439 w444 w449 w454 w459 w464 w469 w474 w478 w482 w488 w493 w498 w500 w502 w507] -> w434
      event "Start": Value Change {
        n119 = event-data() -> ()  [unwired: 1 in, 1 out]
        n120 = call-poly "Enqueue Message.vi"("Message"="Start", "Message Queue"=w440) -> ("error out"=w442:errorcluster, "dup Message Queue"=w439:refnum<queue>)  [unwired: 8 in]
      }
      event "Tank Inlet Valve Toggle": Value Change {
        n121 = event-data() -> ("NewVal"=w443:bool)  [unwired: 1 in]
        "INTAKE VALVE POSITION" <- w443
        n122 = call-poly "Enqueue Message.vi"("Message Data"=w443, "Message"="P1.0", "Message Queue"=w445) -> ("error out"=w447:errorcluster, "dup Message Queue"=w444:refnum<queue>)  [unwired: 7 in]
      }
      event "Tank Outlet Valve Toggle": Value Change {
        n123 = event-data() -> ("NewVal"=w448:bool)  [unwired: 1 in]
        "DUT VALVE POSITION" <- w448
        n124 = call-poly "Enqueue Message.vi"("Message Data"=w448, "Message"="P1.1", "Message Queue"=w450) -> ("error out"=w452:errorcluster, "dup Message Queue"=w449:refnum<queue>)  [unwired: 7 in]
      }
      event "DUT Motor Enable": Value Change {
        n125 = event-data() -> ("NewVal"=w453:bool)  [unwired: 1 in]
        n126 = call-poly "Enqueue Message.vi"("Message Data"=w453, "Message"="P1.2", "Message Queue"=w455) -> ("error out"=w457:errorcluster, "dup Message Queue"=w454:refnum<queue>)  [unwired: 7 in]
      }
      event "DUT Motor Direction": Value Change {
        n127 = event-data() -> ("NewVal"=w458:bool)  [unwired: 1 in]
        n128 = call-poly "Enqueue Message.vi"("Message Data"=w458, "Message"="P1.3", "Message Queue"=w460) -> ("error out"=w462:errorcluster, "dup Message Queue"=w459:refnum<queue>)  [unwired: 7 in]
      }
      event "Motor RPM Target": Value Change {
        n129 = event-data() -> ("NewVal"=w463:u16)  [unwired: 1 in]
        n130 = call-poly "Enqueue Message.vi"("Message Data"=w463, "Message"="Set RPM", "Message Queue"=w465) -> ("error out"=w467:errorcluster, "dup Message Queue"=w464:refnum<queue>)  [unwired: 7 in]
      }
      event "VFD Enable": Value Change {
        n131 = event-data() -> ("NewVal"=w468:bool)  [unwired: 1 in]
        n132 = call-poly "Enqueue Message.vi"("Message Data"=w468, "Message"="VFD Enable", "Message Queue"=w470) -> ("error out"=w472:errorcluster, "dup Message Queue"=w469:refnum<queue>)  [unwired: 7 in]
      }
      event "VFD Reset": Value Change {
        n133 = event-data() -> ("NewVal"=w473:bool)  [unwired: 1 in]
        n134 = call-poly "Enqueue Message.vi"("Message Data"=w473, "Message"="VFD Reset", "Message Queue"=w475) -> ("error out"=w477:errorcluster, "dup Message Queue"=w474:refnum<queue>)  [unwired: 7 in]
      }
      event "Durability Config File Path": Value Change {
        n135 = event-data() -> ()  [unwired: 1 in, 1 out]
        n136 = call-poly "Enqueue Message.vi"("Message"="Config File Update", "Message Queue"=w479) -> ("error out"=w481:errorcluster, "dup Message Queue"=w478:refnum<queue>)  [unwired: 8 in]
      }
      event "Clear Chart": Value Change {
        n137 = event-data() -> ()  [unwired: 1 in, 1 out]
        n138 = call-poly "Enqueue Message.vi"("Message"="Clear Chart", "Message Queue"=w483) -> ("error out"=w485:errorcluster, "dup Message Queue"=w482:refnum<queue>)  [unwired: 8 in]
      }
      event "Stop": Value Change {
        n139 = event-data() -> ("NewVal"=w486:bool)  [unwired: 1 in]
        n140 = call-poly "Enqueue Message.vi"("Message"="Stop", "Message Queue"=w490) -> ("error out"=w489:errorcluster, "dup Message Queue"=w488:refnum<queue>)  [unwired: 8 in]
        n141 = call "StopFGV.vi"("STOP"=w486, "Enum"=enum16{"init", "write", "read"}."write") -> ()  [unwired: 8 in, 2 out]
      }
      event Panel Close? {
        # "Send the 'Confirm Quit' message if the user closes the panel of the VI. Discard the event so the 'Confirm Quit' message has a chance to run."
        n142 = event-data() -> ()  [unwired: 1 in, 1 out]
        n143 = call-poly "Enqueue Message.vi"("Priority Message? (F)"=TRUE, "Message"="Confirm Quit", "Message Queue"=w497) -> ("error out"=w492:errorcluster, "dup Message Queue"=w493:refnum<queue>)  [unwired: 7 in]
        n144 = event-data("Discard?"=TRUE) -> ()  [unwired: 1 in, 1 out]
      }
      event Application Instance Close {
        n145 = event-data() -> ()  [unwired: 1 in, 1 out]
      }
      event Timeout {
        n146 = event-data() -> ()  [unwired: 1 in, 1 out]
        n147 = call-poly "Enqueue Message.vi"("Message"="Monitor VFD", "Message Queue"=w501) -> ("dup Message Queue"=w500:refnum<queue>)  [unwired: 8 in, 1 out]
      }
      event "Exit": Value Change; Panel Close {
        w504 = TRUE  # Priority Message
        # "The UI Message Loop handles sending the Exit message to other loops."
        n148 = event-data() -> ()  [unwired: 1 in, 1 out]
        n149 = call-poly "Enqueue Message.vi"("Priority Message? (F)"=w504, "Message"="Exit", "Message Queue"=w503) -> ("error out"=w506:errorcluster, "dup Message Queue"=w502:refnum<queue>)  [unwired: 7 in]
      }
      event User Event {
        # "The Message Handling Loop processed an \"Exit\" message, which fired this event to stop the Event Handling Loop."
        n150 = event-data() -> ()  [unwired: 1 in, 1 out]
        n151 = local write "Status"("Exit" ("Exit String")) -> ()
      }
    }
    n152 = call "Error Handler - Event Handling Loop.vi"("error in (no error)"=w433, "Message Queue"=w434) -> ("dup error in"=w432:errorcluster)  [unwired: 8 in, 1 out]
  }
  n153 = call "Acquisition Message Loop.vi"("error in (no error)"=w5, "data queue in"=w7, "notifier out"=w9, "Message Queues"=w6) -> ("error out"=w24:errorcluster)  [unwired: 7 in]
  n154 = call "Control Loop.vi"("error in (no error)"=w5, "notifier out"=w9, "Message Queues"=w6) -> ("error out"=w13:errorcluster)  [unwired: 8 in]
  n155 = while "Data Display Loop" {
    tunnel: w9 -> [w524]
    stop <- w523 stop-if-true
    # "Data Display Loop"
    n156 = Wait on Notification(notifier=w524) -> (notification=w522:T4, error out=w523:errorcluster)  [unwired: 3 in, 2 out]
    n157 = global read "TestCaseTimer.vi" "Test State Timer"() -> (→"Test State Timer":dbl)
    n158 = Unbundle By Name(w522) -> ("Waveform Chart Data"=→"Waveform Chart":T5, "Ai0"=→"Tank Pressure (psi)":dbl, "Ai1"=→"DUT Pressure (psi)":dbl, "Ai2"=→"DUT Temp (F)":dbl, "Ai3"=→"Ambent Temp (F)":dbl, "Ai4"=→"Drive Motor RPM":dbl, "Ai5"=→"DUT Pulley RPM":dbl, "Ai6"=→"Air Flow (LPM)":dbl, "Ai7"=→"DUT Motor Current (A)":dbl, "Live Pulley Ratio"=→"Live Pulley Ratio":dbl, "Belt Slip?"=→"Belt Monitor":bool)
  }
  n159 = call "VFD Control Loop.vi"("error in (no error)"=w5, "VFD Notifier"=w1, "Message Queues"=w6) -> ("error out"=w4:errorcluster)  [unwired: 8 in]
  n160 = while {
    tunnel: w1 -> [w531]
    stop <- w532 stop-if-true
    # "VFD Display Data"
    n161 = Wait on Notification(notifier=w531) -> (notification=w530:T1, error out=w532:errorcluster)  [unwired: 3 in, 2 out]
    n162 = Unbundle By Name(w530) -> ("Voltage"=→"Voltage (V)":dbl, "Current"=→"Current (A)":dbl, "Motor Speed"=→"Speed (RPM)":dbl, "Fault"=→"VFD Fault?":bool, "Fault Messages"=→"Fault Messages":string[])
  }
  n163 = call "Logging Message Loop.vi"("error in (no error)"=w5, "data queue in"=w7, "Message Queues"=w6) -> ("error out"=w11:errorcluster)  [unwired: 8 in]
  n164 = global write "Abort.vi" "Abort"(FALSE ("Abort Calibration")) -> ()
  n165 = Unregister For Events(event registration refnum=w21, error in=w28) -> (error out=w22:errorcluster)
  n166 = Merge Errors(w22, w29, w24, w13, w11, w4) -> (w27:errorcluster)
  n167 = call "Destroy User Event - Stop.vi"("error in (no error)"=w27, "User Event - Stop"=w25) -> ("error out"=w16:errorcluster)  [unwired: 9 in]
  n168 = disable-structure shown="Default" {
    disable-tunnel: w16 -> [_ _]
    frame condition #0 {
      # "Call Quit LabVIEW if running as a built application."
      n169 = Quit LabVIEW() -> ()  [unwired: 1 in]
    }
    frame condition #1 (active) {
    }
  }
